vi "校准设置页.vi"() -> ()   [LabVIEW 2016]
uses:
  <vilib>/Analysis/6fits.llb/Curve Fitting Criteria.ctl
  <vilib>/Analysis/NI_AALPro.lvlib
  <vilib>/ptbypt/NI_PtbyPt.lvlib
panel:
  in  "历史数据导入":T1(radio)
  out "校准任务":bool
  in  "二次方程2":cluster{"x^2":dbl, "K":dbl, "B":dbl}
  in  "公式切换阈值滴定数(0~9999)":dbl
  out "校准状态":T2(ring)
  out "模型刷新":bool
  in  "校准按钮":T1(radio)
  in  "校准导入":bool
  in  "曲线模型":T3={"标液浓度1"=0.0, "测量吸光度1"=0.0, "样品1启用"=FALSE, "标液浓度2"=0.0, "测量吸光度2"=0.0, "样品2启用"=FALSE, "标液浓度3"=0.0, "测量吸光度3"=0.0, "样品3启用"=FALSE, "标液浓度4"=0.0, "测量吸光度4"=0.0, "样品4启用"=FALSE, "标液浓度5"=0.0, "测量吸光度5"=0.0, "样品5启用"=FALSE, "模型"=enum."线性", "精度"=4.0, "XY图"=[], "拟合公式"="", "r^2"=0.0, "标样一校准时间"=timestamp(0 s since 1904-01-01), "标样二校准时间"=timestamp(0 s since 1904-01-01), "标样三校准时间"=timestamp(0 s since 1904-01-01), "标样四校准时间"=timestamp(0 s since 1904-01-01), "标样五校准时间"=timestamp(0 s since 1904-01-01), "二次方程"={"x^2"=0.0, "K"=0.0, "B"=0.0}, "标定时间"=timestamp(0 s since 1904-01-01), "拟合公式 2"="", "r^2 2"=0.0} {"r^2 2" format="%.7f"; "标定时间" format="%<%Y/%m/%d %H:%M:%S>T"; "标样五校准时间" format="%<%Y/%m/%d %H:%M:%S>T"; "标样四校准时间" format="%<%Y/%m/%d %H:%M:%S>T"; "标样三校准时间" format="%<%Y/%m/%d %H:%M:%S>T"; "标样二校准时间" format="%<%Y/%m/%d %H:%M:%S>T"; "标样一校准时间" format="%<%Y/%m/%d %H:%M:%S>T"; "r^2" format="%.7f"; "测量吸光度5" format="%#.6f"; "测量吸光度4" format="%#.6f"; "测量吸光度3" format="%#.6f"; "测量吸光度2" format="%#.6f"; "测量吸光度1" format="%#.6f"}
  in  "测量模式":T4(ring)
  in  "参数下拉列表":u16(ring)=1 items=["挥发酚"=1]
  in  "量程下拉列表":enum16{"低量程", "高量程"}(ring)
  # "校准时间"
  # "标液浓度"
  # "滴定数"
  # "标液一"
  # "标液二"
  # "标液三"
  # "零点"
  # "跨度"
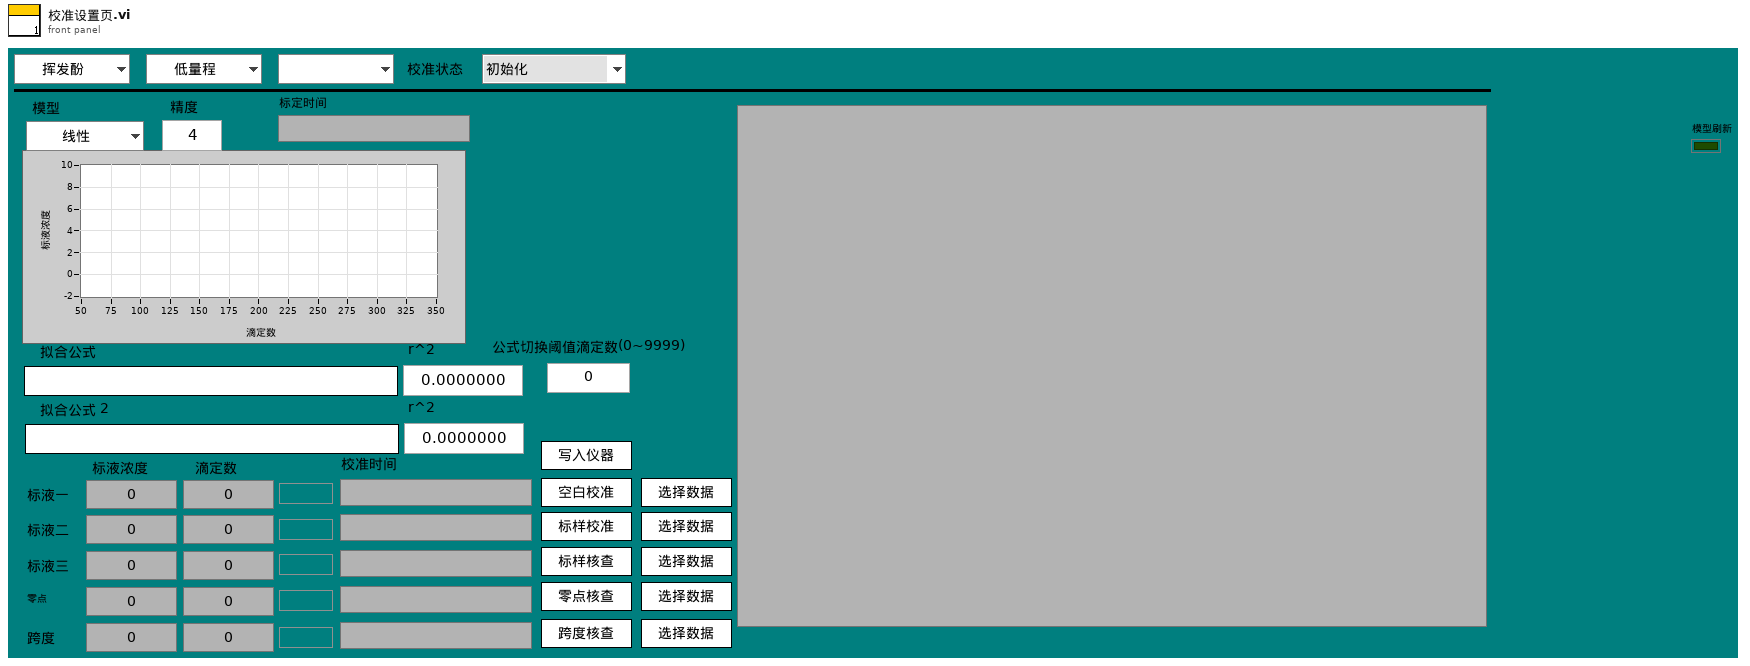
[diagram p1: front panel]
types:
  T1 = enum32{"未选择", "空白校准", "标样校准", "标样核查", "零点核查", "跨度核查"}
  T2 = enum16{"初始化", "解析数据", "判断任务类型", "执行测试任务", "等待测试任务完成", "获取测试数据", "任务结束判定", "计算公式", "结束"}
  T3 = cluster{"标液浓度1":dbl, "测量吸光度1":dbl, "样品1启用":bool, "标液浓度2":dbl, "测量吸光度2":dbl, "样品2启用":bool, "标液浓度3":dbl, "测量吸光度3":dbl, "样品3启用":bool, "标液浓度4":dbl, "测量吸光度4":dbl, "样品4启用":bool, "标液浓度5":dbl, "测量吸光度5":dbl, "样品5启用":bool, "模型":enum32{"线性", "多项式", "折线"}, "精度":dbl, "XY图":cluster{"X Values":dbl[], "Y Values":dbl[]}[], "拟合公式":string, "r^2":dbl, "标样一校准时间":timestamp, "标样二校准时间":timestamp, "标样三校准时间":timestamp, "标样四校准时间":timestamp, "标样五校准时间":timestamp, "二次方程":cluster{"x^2":dbl, "K":dbl, "B":dbl}, "标定时间":timestamp, "拟合公式 2":string, "r^2 2":dbl}
  T4 = enum16{"", "水样测量", "标样核查", "零点核查", "跨度核查", "空白测试", "平行样测试", "加标回收", "空白校准", "标样校准"}
  T5 = typedef "校准任务.ctl" = cluster{"id":u16, "任务类型":enum16{"未选择", "空白校准", "标样校准", "标样核查", "零点核查", "跨度核查"}, "量程下拉列表":enum16{"低量程", "高量程"}, "状态":enum16{"已执行", "待执行", "执行中", "停止"}, "标液浓度":dbl, "吸光值":dbl, "校准时间":timestamp, "报警状态":enum16{"正常数据", "报警数据"}}
  T6 = enum16{"", "水样测量", "标样核查", "零点核查", "跨度核查", "空白测试", "平行样测试", "加标回收"}
  T7 = cluster{"标液浓度1":dbl, "测量吸光度1":dbl, "样品1启用":bool, "标液浓度2":dbl, "测量吸光度2":dbl, "样品2启用":bool, "标液浓度3":dbl, "测量吸光度3":dbl, "样品3启用":bool, "标液浓度4":dbl, "测量吸光度4":dbl, "样品4启用":bool, "标液浓度5":dbl, "测量吸光度5":dbl, "样品5启用":bool, "模型":enum32{"线性", "多项式", "折线"}, "精度":dbl, "XY图":cluster{"X Values":dbl[], "Y Values":dbl[]}[], "拟合公式":string, "r^2":dbl, "标样一校准时间":timestamp, "标样二校准时间":timestamp, "标样三校准时间":timestamp, "标样四校准时间":timestamp, "标样五校准时间":timestamp, "二次方程":cluster{"c":dbl, "x":dbl, "x^2":dbl}, "标定时间":timestamp, "拟合公式 2":string, "r^2 2":dbl}[][]
  T8 = cluster{"标液浓度1":dbl, "测量吸光度1":dbl, "样品1启用":bool, "标液浓度2":dbl, "测量吸光度2":dbl, "样品2启用":bool, "标液浓度3":dbl, "测量吸光度3":dbl, "样品3启用":bool, "标液浓度4":dbl, "测量吸光度4":dbl, "样品4启用":bool, "标液浓度5":dbl, "测量吸光度5":dbl, "样品5启用":bool, "模型":enum32{"线性", "多项式", "折线"}, "精度":dbl, "XY图":cluster{"X Values":dbl[], "Y Values":dbl[]}[], "拟合公式":string, "r^2":dbl, "标样一校准时间":timestamp, "标样二校准时间":timestamp, "标样三校准时间":timestamp, "标样四校准时间":timestamp, "标样五校准时间":timestamp, "二次方程":cluster{"c":dbl, "x":dbl, "x^2":dbl}, "标定时间":timestamp, "拟合公式 2":string, "r^2 2":dbl}
  T9 = typedef "NI_AALPro.lvlib/Curve Fitting Criteria.ctl" = u16
  T10 = enum32{"Bad", "Idle", "Run top level", "Running"}
  T11 = cluster{"时间":timestamp, "标液值":dbl, "检测值":dbl, "吸光值":dbl}
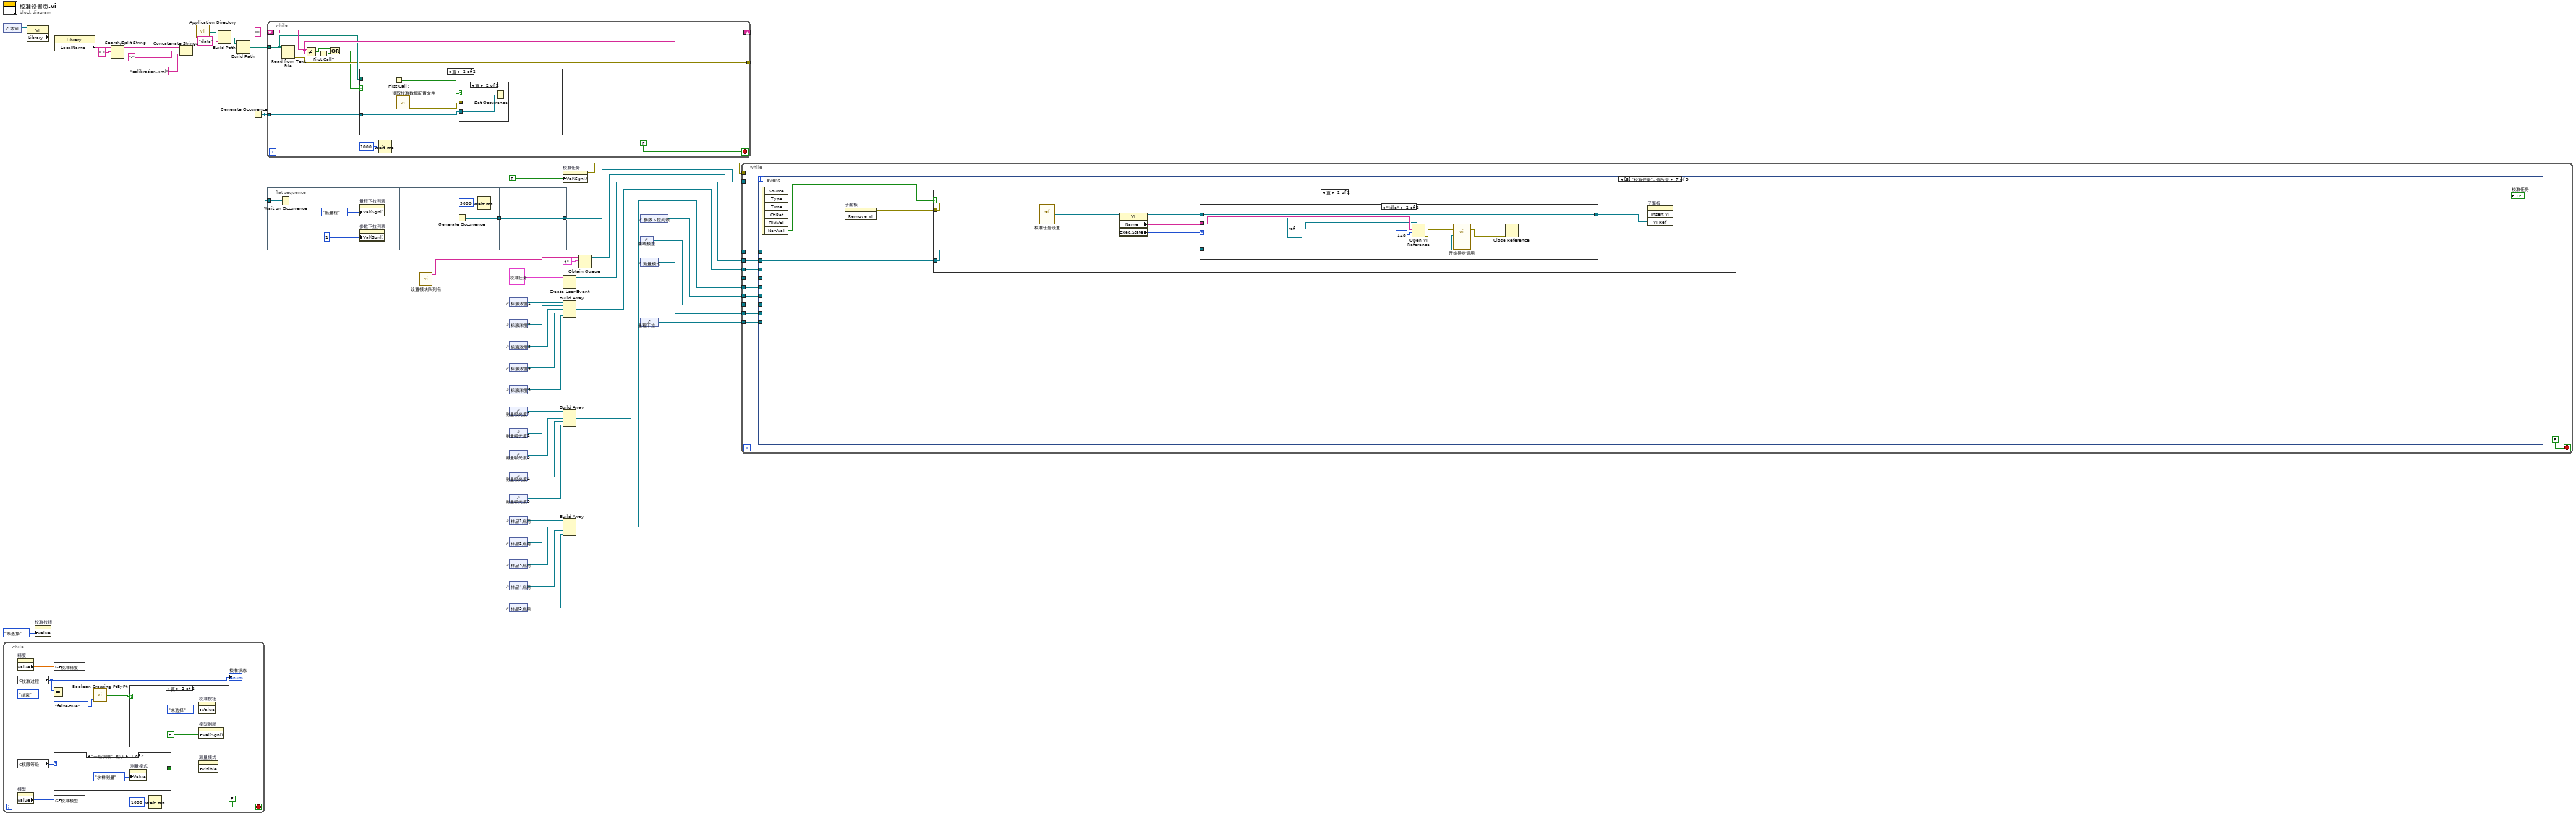
[diagram p0: block diagram]
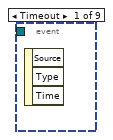
[diagram p4: hidden frame]
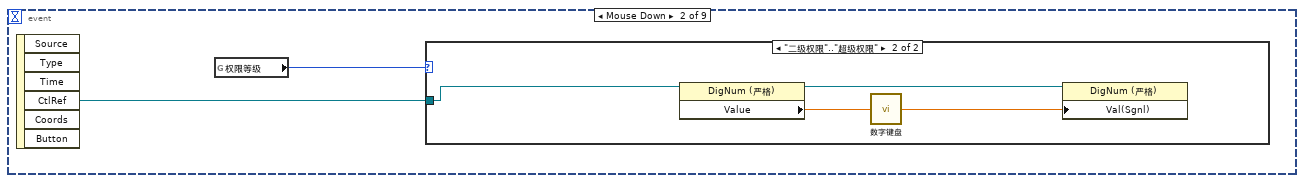
[diagram p5: hidden frame]
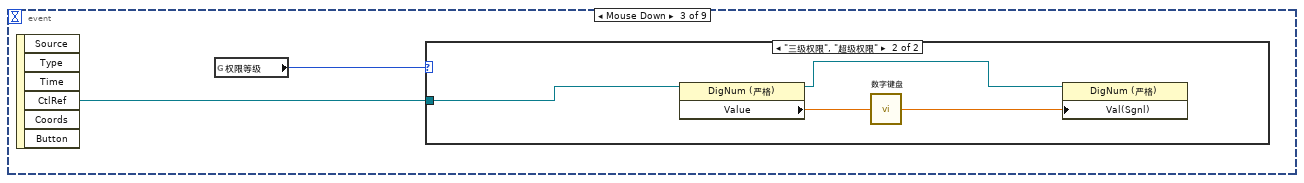
[diagram p7: hidden frame]
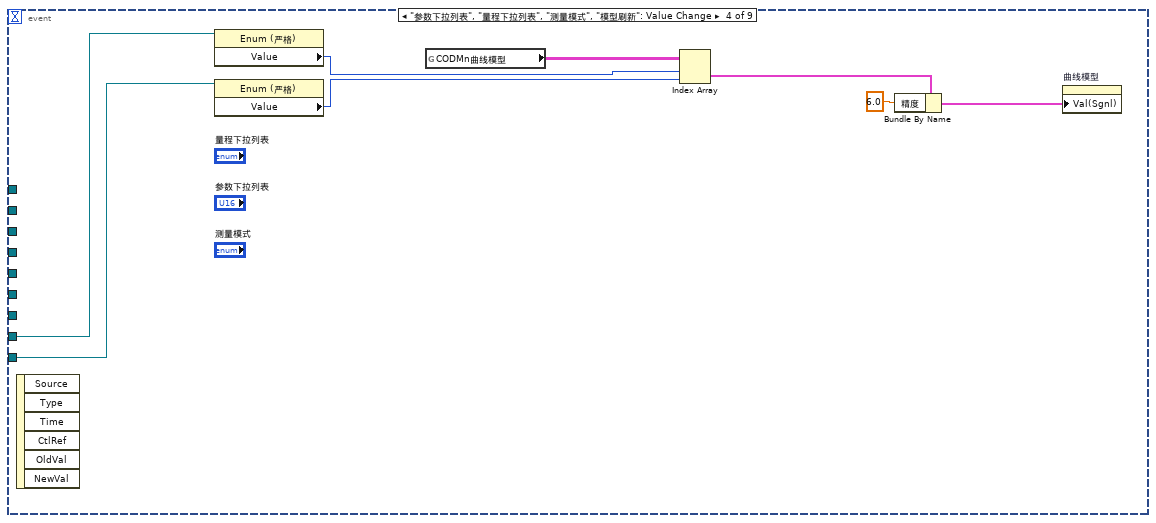
[diagram p9: hidden frame]
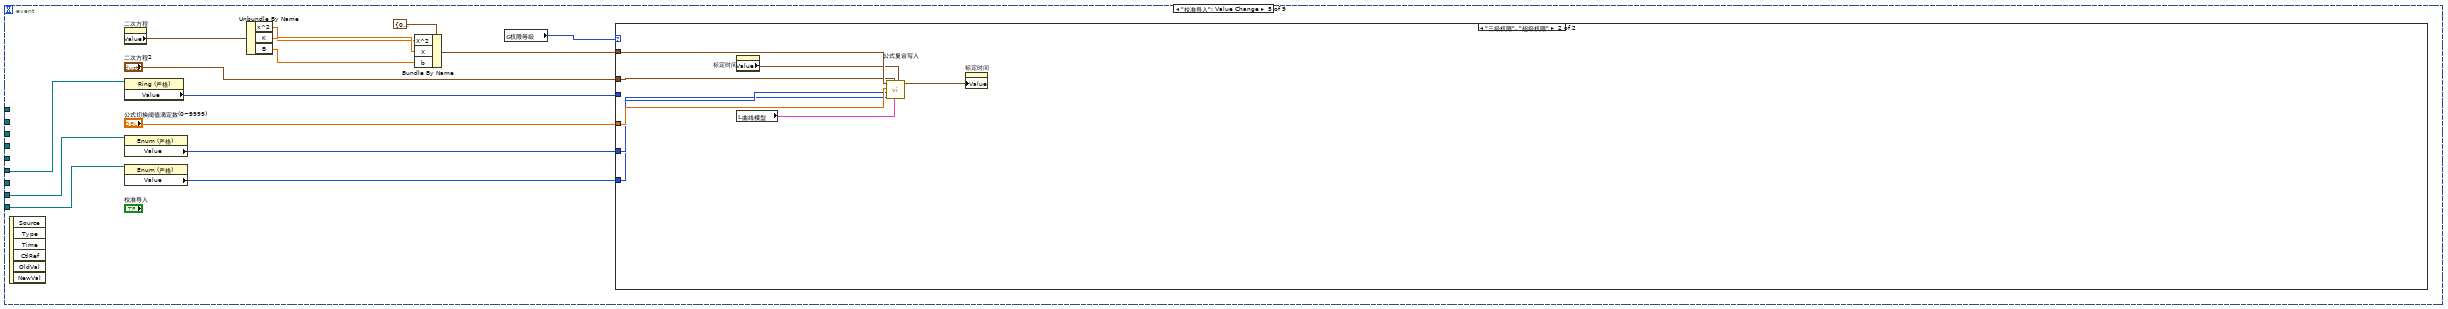
[diagram p10: hidden frame]
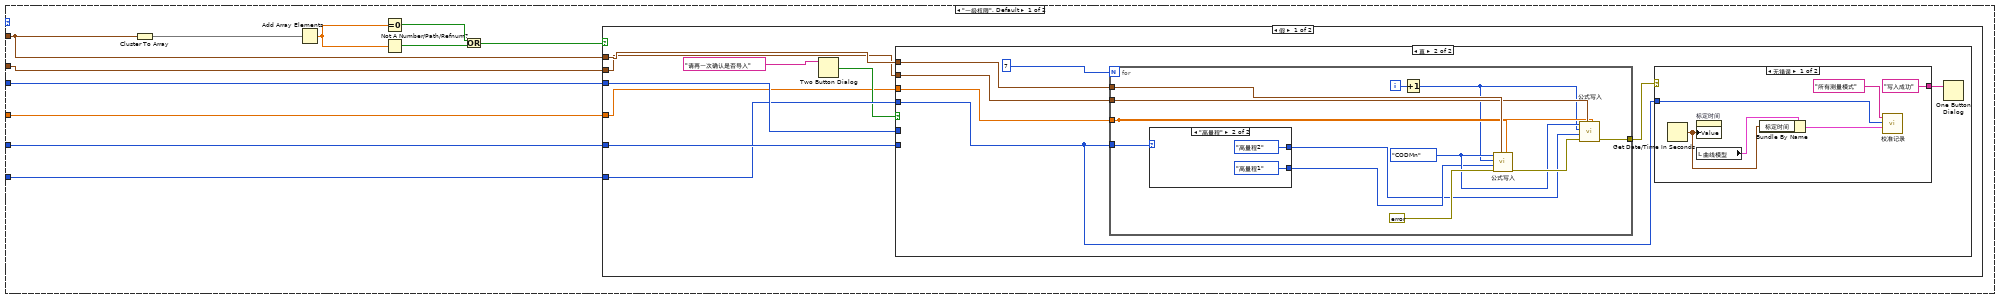
[diagram p11: hidden frame]
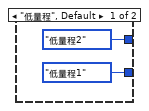
[diagram p13: hidden frame]
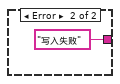
[diagram p14: hidden frame]
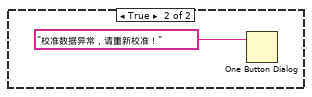
[diagram p15: hidden frame]
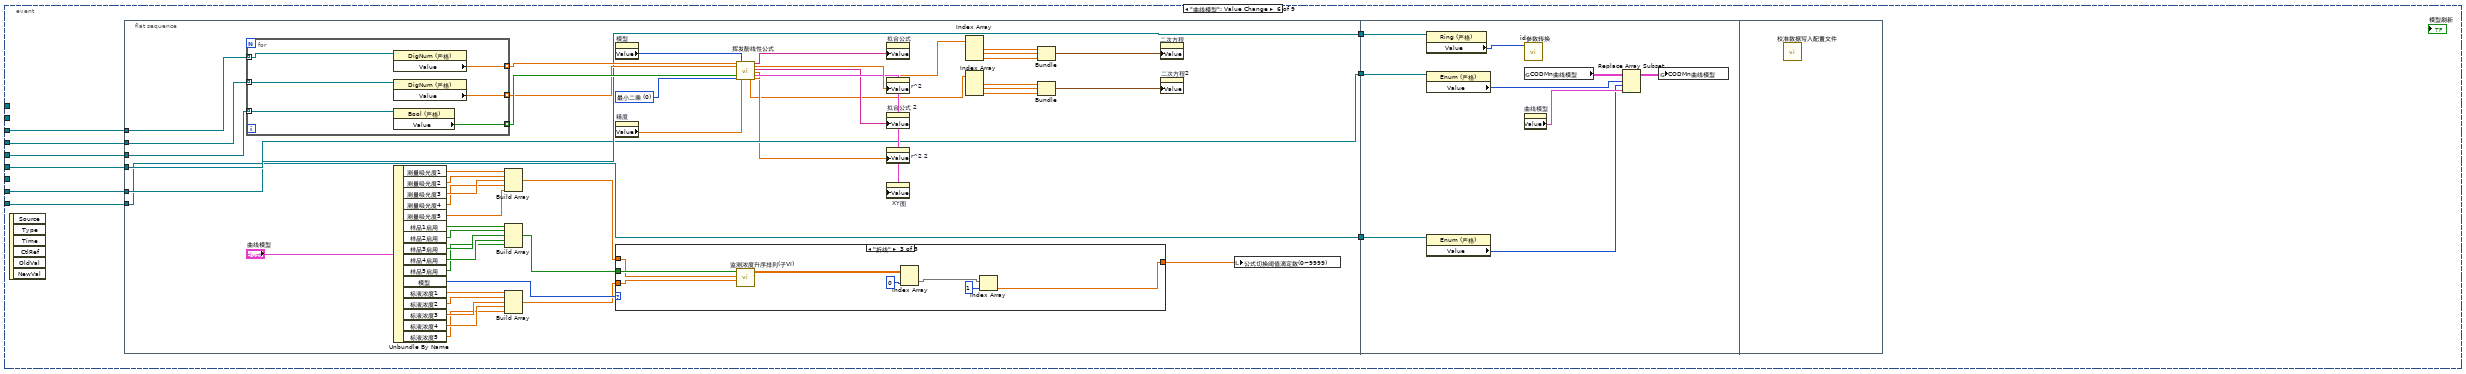
[diagram p16: hidden frame]
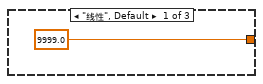
[diagram p17: hidden frame]
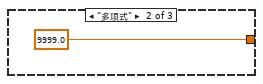
[diagram p18: hidden frame]
diagram:
  n1 = control-ref of="本VI"() -> (w8:refnum<vi>)
  n2 = while {
    stop <- FALSE stop-if-true
    n3 = property on="精度" class="DigNum (严格)"() -> ("Value"=w47:dbl)  [unwired: 2 in, 2 out]
    n4 = global read "VAR挥发酚全局变量.vi" "校准过程"() -> (w49:T2)
    "校准状态" <- w49
    n5 = global read "VAR挥发酚全局变量.vi" "权限等级"() -> (w55:enum16{"一级权限", "二级权限", "三级权限", "超级权限"})
    n6 = property on="模型" class="Enum (严格)"() -> ("Value"=w48:enum32{"线性", "多项式", "折线"})  [unwired: 2 in, 2 out]
    n7 = Equal?(x=w49, y=T2."结束" ("校准过程")) -> (x = y?=w53:bool)
    n8 = global write "VAR挥发酚全局变量.vi" "校准精度"(w47) -> ()
    n9 = case shown="\"一级权限\", 默认" w55 {
      tunnel: [_ TRUE ("可见")] -> w54
      frame "一级权限", Default {
        n10 = property on="测量模式" class="Enum (严格)"("Value"=T6."水样测量" ("测量模式")) -> ()  [unwired: 2 in, 2 out]
      }
      frame "三级权限", "超级权限" {
      }
    }
    n11 = global write "VAR挥发酚全局变量.vi" "校准模型"(w48) -> ()
    n12 = call <vilib>:"Boolean Crossing PtByPt.vi"("direction"=enum16{"either", "false-true", "true-false"}."false-true", "input"=w53) -> ("crossing"=w51:bool)  [unwired: 1 in]
    n13 = case shown="真" w51 {
      frame False {
      }
      frame True {
        n14 = property on="校准按钮" class="RadioBtnsControl (严格)"("Value"=T1."未选择" ("校准按钮")) -> ()  [unwired: 2 in, 2 out]
        n15 = property on="模型刷新" class="Bool (严格)"("Val(Sgnl)"=FALSE ("值(信号)")) -> ()  [unwired: 2 in, 2 out]
      }
    }
    n16 = Wait (ms)(milliseconds to wait=u32 1000 ("等待时间（毫秒）")) -> ()  [unwired: 1 out]
    n17 = property on="测量模式" class="Enum (严格)"("Visible"=w54) -> ()  [unwired: 2 in, 2 out]
  }
  n18 = property class="VI"(reference=w8) -> ("Library"=w17:refnum<vi>)  [unwired: 1 in, 2 out]
  n19 = property on="校准按钮" class="RadioBtnsControl (严格)"("Value"=T1."未选择" ("校准按钮")) -> ()  [unwired: 2 in, 2 out]
  n20 = property class="Library"(reference=w17) -> ("LocalName"=w15:string)  [unwired: 1 in, 2 out]
  n21 = Search/Split String(string=w15, search string/char (-)="." ("搜索字符串/字符(-)")) -> (substring before match=w13:string)  [unwired: 1 in, 2 out]
  n22 = Concatenate Strings(w13, "-" ("字符串"), "calibration.xml" ("名称或相对路径")) -> (w10:string)
  n23 = call <vilib>:"Application Directory.vi"() -> ("Application Directory"=w18:path)
  n24 = Build Path(base path=w18, name or relative path="data" ("名称或相对路径")) -> (appended path=w16:path)
  n25 = Build Path(base path=w16, name or relative path=w10) -> (appended path=w9:path)
  n26 = Generate Occurrence() -> (w6:refnum<k4>)
  n27 = while {
    shift-right: [w69] -> _
    shift-left: "" -> [w70]
    tunnel: w9 -> [w68]
    tunnel: [w66] -> _
    tunnel: w6 -> [w62]
    stop <- FALSE stop-if-true
    n28 = Read from Text File(file (use dialog)=w68) -> (text=w69:string, error out=w66:errorcluster)  [unwired: 3 in, 2 out]
    n29 = Not Equal?(x=w70, y=w69) -> (x != y?=w64:bool)
    n30 = First Call?() -> (First Call?: T/F=w65:bool)
    n31 = Or(x=w64, y=w65) -> (x .or. y?=w63:bool)
    n32 = case shown="真" w63 {
      tunnel: w68 -> [_ _]
      tunnel: w62 -> [_ w73]
      frame False {
      }
      frame True {
        n33 = First Call?() -> (First Call?: T/F=w74:bool)
        n34 = call "读取校准数据配置文件.vi"() -> ("错误输出"=w72:errorcluster)  [unwired: 11 in]
        n35 = case shown="真" w74 {
          tunnel: w73 -> [_ w75]
          tunnel: w72 -> [_ _]
          frame False {
          }
          frame True {
            n36 = Set Occurrence(w75) -> ()
          }
        }
      }
    }
    n37 = Wait (ms)(milliseconds to wait=u32 1000 ("等待时间（毫秒）")) -> ()  [unwired: 1 out]
  }
  n38 = flat-sequence {
    tunnel: w6 -> [w76]
    tunnel: [w80] -> w46
    tunnel: [w81] -> w45
    tunnel: w46 -> [w81]
    frame #0 {
      n39 = Wait on Occurrence(2:w76) -> ()  [unwired: 2 in, 1 out]
    }
    frame #1 {
      n40 = property on="量程下拉列表" class="Enum (严格)"("Val(Sgnl)"=enum16{"低量程", "高量程"}."低量程" ("值(信号)")) -> ()  [unwired: 2 in, 2 out]
      n41 = property on="参数下拉列表" class="Ring (严格)"("Val(Sgnl)"=u16 1 ("值(信号)")) -> ()  [unwired: 2 in, 2 out]
    }
    frame #2 {
      n42 = Generate Occurrence() -> (w80:refnum<k4>)
      n43 = Wait (ms)(milliseconds to wait=u32 5000 ("等待时间（毫秒）")) -> ()  [unwired: 1 out]
    }
    frame #3 {
    }
  }
  n44 = call "设置模块队列名.vi"() -> ("Msg"=w1:string)  [unwired: 11 in]
  n45 = control-ref of="标液浓度1"() -> (w31:refnum<vi>)
  n46 = control-ref of="标液浓度2"() -> (w30:refnum<vi>)
  n47 = control-ref of="标液浓度3"() -> (w29:refnum<vi>)
  n48 = control-ref of="标液浓度4"() -> (w28:refnum<vi>)
  n49 = control-ref of="标液浓度5"() -> (w27:refnum<vi>)
  n50 = control-ref of="测量吸光度1"() -> (w33:refnum<vi>)
  n51 = control-ref of="测量吸光度2"() -> (w34:refnum<vi>)
  n52 = control-ref of="测量吸光度3"() -> (w35:refnum<vi>)
  n53 = control-ref of="测量吸光度4"() -> (w36:refnum<vi>)
  n54 = control-ref of="测量吸光度5"() -> (w37:refnum<vi>)
  n55 = control-ref of="样品1启用"() -> (w43:refnum<vi>)
  n56 = control-ref of="样品2启用"() -> (w42:refnum<vi>)
  n57 = control-ref of="样品3启用"() -> (w41:refnum<vi>)
  n58 = control-ref of="样品4启用"() -> (w40:refnum<vi>)
  n59 = control-ref of="样品5启用"() -> (w39:refnum<vi>)
  n60 = property on="校准任务" class="Bool (严格)"("Val(Sgnl)"=TRUE ("值(信号)")) -> (error out=w4:errorcluster)  [unwired: 2 in, 1 out]
  n61 = Create User Event(user event datatype=T5 {"id"=0, "任务类型"=enum."未选择", "量程下拉列表"=enum."低量程", "状态"=enum."已执行", "标液浓度"=0.0, "吸光值"=0.0, "校准时间"=timestamp(0 s since 1904-01-01), "报警状态"=enum."正常数据"} ("校准任务")) -> (user event=w2:refnum<user-event>)  [unwired: 1 in, 1 out]
  n62 = Build Array(w31, w30, w29, w28, w27) -> (w26:refnum<vi>[])
  n63 = Build Array(w33, w34, w35, w36, w37) -> (w32:refnum<vi>[])
  n64 = Build Array(w43, w42, w41, w40, w39) -> (w38:refnum<vi>[])
  n65 = Obtain Queue(name (unnamed)=w1, element data type=cluster{"命令":string, "data":variant} {"命令"="", "data"=variant}) -> (queue out=w22:refnum<queue>)  [unwired: 3 in, 2 out]
  n66 = control-ref of="参数下拉列表"() -> (w44:refnum<vi>)
  n67 = control-ref of="曲线模型"() -> (w20:refnum<vi>)
  n68 = control-ref of="测量模式"() -> (w25:refnum<vi>)
  n69 = control-ref of="量程下拉列表"() -> (w24:refnum<vi>)
  n70 = while {
    tunnel: w45 -> [_]
    tunnel: w44 -> [w90]
    tunnel: w38 -> [w89]
    tunnel: w32 -> [w88]
    tunnel: w26 -> [w87]
    tunnel: w25 -> [w86]
    tunnel: w24 -> [w85]
    tunnel: w22 -> [w84]
    tunnel: w20 -> [w83]
    tunnel: w4 -> [_]
    tunnel: w2 -> [w82]
    stop <- FALSE stop-if-true
    n71 = event shown="[6] \"校准任务\": 值改变" {
      selector: _ -> [_ _ _ _ _ _ _ _ _]
      dyn-events: _ -> [_ _ _ _ _ _ _ _ _]
      timeout: _ -> [_ _ _ _ _ _ _ _ _]
      tunnel: w90 -> [_ _ _ _ w126 w189 _ w295 w323]
      tunnel: w89 -> [_ _ _ _ _ w193 _ _ _]
      tunnel: w88 -> [_ _ _ _ _ w192 _ _ _]
      tunnel: w87 -> [_ _ _ _ _ w191 _ _ _]
      tunnel: w86 -> [_ _ _ w111 w124 w187 _ w290 w318]
      tunnel: w85 -> [_ _ _ w110 w122 w185 _ w294 w322]
      tunnel: w84 -> [_ _ _ _ _ _ _ w296 w324]
      tunnel: w83 -> [_ _ _ _ _ _ _ w288 _]
      tunnel: w82 -> [_ _ _ _ _ _ w268 w287 w317]
      event Timeout {
        n72 = event-data() -> ()  [unwired: 1 in, 3 out]
      }
      event "曲线模型.标液浓度1", "曲线模型.标液浓度2", "曲线模型.标液浓度3", "曲线模型.标液浓度4", "曲线模型.标液浓度5", "曲线模型.精度": Mouse Down {
        n73 = event-data() -> ("CtlRef"=w93:refnum<vi>)  [unwired: 1 in, 5 out]
        n74 = global read "VAR挥发酚全局变量.vi" "权限等级"() -> (w92:enum16{"一级权限", "二级权限", "三级权限", "超级权限"})
        n75 = case shown="\"二级权限\"..\"超级权限\"" w92 {
          tunnel: w93 -> [_ w97]
          frame "一级权限", Default {
          }
          frame "二级权限".."超级权限" {
            n76 = property class="DigNum (严格)"(reference=w97) -> (reference out=w95:refnum<vi>, "Value"=w96:dbl)  [unwired: 1 in, 1 out]
            n77 = call "数字键盘.vi"("OldNumber"=w96) -> ("NewNumber"=w94:dbl)
            n78 = property class="DigNum (严格)"(reference=w95, "Val(Sgnl)"=w94) -> ()  [unwired: 1 in, 2 out]
          }
        }
      }
      event "曲线模型.测量吸光度1", "曲线模型.测量吸光度2", "曲线模型.测量吸光度3", "曲线模型.测量吸光度4", "曲线模型.测量吸光度5": Mouse Down {
        n79 = event-data() -> ("CtlRef"=w99:refnum<vi>)  [unwired: 1 in, 5 out]
        n80 = global read "VAR挥发酚全局变量.vi" "权限等级"() -> (w98:enum16{"一级权限", "二级权限", "三级权限", "超级权限"})
        n81 = case shown="\"三级权限\", \"超级权限\"" w98 {
          tunnel: w99 -> [_ w103]
          frame "一级权限", Default {
          }
          frame "三级权限", "超级权限" {
            n82 = property class="DigNum (严格)"(reference=w103) -> (reference out=w101:refnum<vi>, "Value"=w102:dbl)  [unwired: 1 in, 1 out]
            n83 = call "数字键盘.vi"("OldNumber"=w102) -> ("NewNumber"=w100:dbl)
            n84 = property class="DigNum (严格)"(reference=w101, "Val(Sgnl)"=w100) -> ()  [unwired: 1 in, 2 out]
          }
        }
      }
      event "参数下拉列表", "量程下拉列表", "测量模式", "模型刷新": Value Change {
        n85 = event-data() -> ()  [unwired: 1 in, 6 out]
        n86 = property class="Enum (严格)"(reference=w111) -> ("Value"=w108:T4)  [unwired: 1 in, 2 out]
        n87 = property class="Enum (严格)"(reference=w110) -> ("Value"=w107:enum16{"低量程", "高量程"})  [unwired: 1 in, 2 out]
        n88 = global read "校准数据全局变量.vi" "CODMn曲线模型"() -> (w109:T7)
        n89 = Index Array(array=w109, index (row)=w108, index (col)=w107) -> (element=w106:T8)
        n90 = Bundle By Name(cluster=w106, "精度"=6.0 ("值")) -> (w105:T8)
        n91 = property on="曲线模型" class="Clust (严格)"("Val(Sgnl)"=w105) -> ()  [unwired: 2 in, 2 out]
      }
      event "校准导入": Value Change {
        n92 = event-data() -> ()  [unwired: 1 in, 6 out]
        n93 = property on="二次方程" class="Clust (严格)"() -> ("Value"=w116:cluster{"x^2":dbl, "K":dbl, "B":dbl})  [unwired: 2 in, 2 out]
        n94 = property class="Ring (严格)"(reference=w126) -> ("Value"=w125:u16)  [unwired: 1 in, 2 out]
        n95 = property class="Enum (严格)"(reference=w124) -> ("Value"=w123:T4)  [unwired: 1 in, 2 out]
        n96 = property class="Enum (严格)"(reference=w122) -> ("Value"=w121:enum16{"低量程", "高量程"})  [unwired: 1 in, 2 out]
        n97 = Unbundle By Name(w116) -> ("x^2"=w117:dbl, "K"=w118:dbl, "B"=w119:dbl)
        n98 = Bundle By Name(cluster=cluster{"X^2":dbl, "X":dbl, "b":dbl} {"X^2"=0.0, "X"=0.0, "b"=0.0} ("公式"), "X^2"=w117, "X"=w118, "b"=w119) -> (w115:cluster{"X^2":dbl, "X":dbl, "b":dbl})
        n99 = global read "VAR挥发酚全局变量.vi" "权限等级"() -> (w120:enum16{"一级权限", "二级权限", "三级权限", "超级权限"})
        n100 = case shown="\"三级权限\", \"超级权限\"" w120 {
          tunnel: w125 -> [w137 _]
          tunnel: w123 -> [w136 w182]
          tunnel: w121 -> [w135 w181]
          tunnel: w115 -> [w129 w184]
          tunnel: "公式切换阈值滴定数(0~9999)" -> [w128 w183]
          tunnel: "二次方程2" -> [w127 w180]
          frame "一级权限", Default {
            n101 = Cluster To Array(cluster=w129) -> (array=w134:dbl[])
            n102 = Add Array Elements(numeric array=w134) -> (sum=w133:dbl)
            n103 = Equal To 0?(x=w133) -> (x = 0?=w131:bool)
            n104 = Not A Number/Path/Refnum?(number/path/refnum=w133) -> (NaN/Path/Refnum?=w132:bool)
            n105 = Or(x=w131, y=w132) -> (x .or. y?=w130:bool)
            n106 = case shown="假" w130 {
              tunnel: w137 -> [w145 _]
              tunnel: w136 -> [w144 _]
              tunnel: w135 -> [w143 _]
              tunnel: w129 -> [w140 _]
              tunnel: w128 -> [w139 _]
              tunnel: w127 -> [w138 _]
              frame False {
                n107 = Two Button Dialog(message="请再一次确认是否导入" ("消息")) -> (T button?=w141:bool)  [unwired: 2 in]
                n108 = case shown="真" w141 {
                  tunnel: w145 -> [_ _]
                  tunnel: w144 -> [_ _]
                  tunnel: w143 -> [_ w146]
                  tunnel: w140 -> [_ w151]
                  tunnel: w139 -> [_ w148]
                  tunnel: w138 -> [_ w149]
                  frame False {
                  }
                  frame True {
                    n109 = for {
                      N: 7 -> [_]
                      tunnel: w151 -> [w163]
                      tunnel: [w161] -> w150
                      tunnel: w149 -> [w160]
                      tunnel: w148 -> [w159]
                      tunnel: w146 -> [w157]
                      i -> [w154]
                      w158 = enum16{"CODMn"}."CODMn" ("测量参数")
                      n110 = case shown="\"高量程\"" w157 {
                        tunnel: [enum16{"低量程1", "低量程2", "高量程1", "高量程2"}."低量程1" ("量程") enum16{"低量程1", "低量程2", "高量程1", "高量程2"}."高量程1" ("量程")] -> w156
                        tunnel: [enum16{"低量程1", "低量程2", "高量程1", "高量程2"}."低量程2" ("量程") enum16{"低量程1", "低量程2", "高量程1", "高量程2"}."高量程2" ("量程")] -> w155
                        frame "低量程", Default {
                        }
                        frame "高量程" {
                        }
                      }
                      n111 = Increment(x=w154) -> (x+1=w153:i32)
                      n112 = call "公式写入.vi"("临界滴定数"=w159, "公式"=w163, "error in (no error)"=errorcluster {"status"=FALSE, "code"=0, "source"=""} ("error out"), "量程"=w156, "测量模式"=w153, "测量参数"=w158) -> ("error out"=w162:errorcluster)  [unwired: 5 in]
                      n113 = call "公式写入.vi"("临界滴定数"=w159, "公式"=w160, "error in (no error)"=w162, "量程"=w155, "测量模式"=w153, "测量参数"=w158) -> ("error out"=w161:errorcluster)  [unwired: 5 in]
                    }
                    n114 = case shown="无错误" w150 {
                      tunnel: ["写入成功" "写入失败"] -> w152
                      tunnel: w146 -> [w173 _]
                      frame No Error {
                        n115 = Get Date/Time In Seconds() -> (seconds since 1Jan1904=w170:timestamp)
                        n116 = property on="标定时间" class="AbsTime (严格)"("Value"=w170) -> ()  [unwired: 2 in, 2 out]
                        n117 = local read "曲线模型"() -> (w171:T3)
                        n118 = Bundle By Name(cluster=w171, "标定时间"=w170) -> (w169:T3)
                        n119 = call "校准记录.vi"("曲线模型"=w169, "量程"=w173, "测量模式"="所有测量模式") -> ()  [unwired: 8 in, 1 out]
                      }
                      frame Error {
                      }
                    }
                    n120 = One Button Dialog(message=w152) -> ()  [unwired: 1 in, 1 out]
                  }
                }
              }
              frame True {
                n121 = One Button Dialog(message="校准数据异常，请重新校准！" ("消息")) -> ()  [unwired: 1 in, 1 out]
              }
            }
          }
          frame "三级权限", "超级权限" {
            n122 = property on="标定时间" class="AbsTime (严格)"() -> ("Value"=w177:timestamp)  [unwired: 2 in, 2 out]
            n123 = local read "曲线模型"() -> (w178:T3)
            n124 = call "公式复合写入.vi"("标定时间输入"=w177, "曲线模型"=w178, "公式 2"=w180, "量程下拉列表"=w181, "测量模式"=w182, "临界滴定数"=w183, "公式"=w184) -> ("标定时间输出"=w179:timestamp)  [unwired: 4 in]
            n125 = property on="标定时间" class="AbsTime (严格)"("Value"=w179) -> ()  [unwired: 2 in, 2 out]
          }
        }
      }
      event "曲线模型": Value Change {
        n126 = event-data() -> ()  [unwired: 1 in, 6 out]
        n127 = flat-sequence {
          tunnel: w193 -> [w241]
          tunnel: w192 -> [w239]
          tunnel: w191 -> [w237]
          tunnel: [w224] -> w190
          tunnel: w189 -> [w224]
          tunnel: [w223] -> w188
          tunnel: w187 -> [w223]
          tunnel: [w222] -> w186
          tunnel: w185 -> [w222]
          tunnel: w190 -> [w266]
          tunnel: w188 -> [w263]
          tunnel: w186 -> [w262]
          frame #0 {
            w233 = T9 0 items=["最小二乘", "最小绝对残差", "Bisquare"] ("method")
            n128 = for {
              tunnel: w241 -> [w257] mode=indexing
              tunnel: [w256] -> w240 mode=indexing
              tunnel: w239 -> [w255] mode=indexing
              tunnel: [w254] -> w238 mode=indexing
              tunnel: w237 -> [w253] mode=indexing
              tunnel: [w252] -> w236 mode=indexing
              n129 = property class="DigNum (严格)"(reference=w253) -> ("Value"=w252:dbl)  [unwired: 1 in, 2 out]
              n130 = property class="DigNum (严格)"(reference=w255) -> ("Value"=w254:dbl)  [unwired: 1 in, 2 out]
              n131 = property class="Bool (严格)"(reference=w257) -> ("Value"=w256:bool)  [unwired: 1 in, 2 out]
            }
            n132 = Unbundle By Name("曲线模型") -> ("测量吸光度1"=w220:dbl, "测量吸光度2"=w219:dbl, "测量吸光度3"=w218:dbl, "测量吸光度4"=w216:dbl, "测量吸光度5"=w217:dbl, "样品1启用"=w215:bool, "样品2启用"=w214:bool, "样品3启用"=w213:bool, "样品4启用"=w212:bool, "样品5启用"=w211:bool, "模型"=w200:enum32{"线性", "多项式", "折线"}, "标液浓度1"=w199:dbl, "标液浓度2"=w198:dbl, "标液浓度3"=w197:dbl, "标液浓度4"=w196:dbl, "标液浓度5"=w195:dbl)
            n133 = Build Array(w220, w219, w218, w216, w217) -> (w209:dbl[])
            n134 = Build Array(w215, w214, w213, w212, w211) -> (w210:bool[])
            n135 = Build Array(w199, w198, w197, w196, w195) -> (w194:dbl[])
            n136 = property on="模型" class="Enum (严格)"() -> ("Value"=w235:enum32{"线性", "多项式", "折线"})  [unwired: 2 in, 2 out]
            n137 = property on="精度" class="DigNum (严格)"() -> ("Value"=w234:dbl)  [unwired: 2 in, 2 out]
            n138 = case shown="\"折线\"" w200 {
              tunnel: w210 -> [_ _ w249]
              tunnel: w209 -> [_ _ w248]
              tunnel: [9999.0 ("数值") 9999.0 ("数值") w250] -> w201
              tunnel: w194 -> [_ _ w247]
              frame "线性", Default {
              }
              frame "多项式" {
              }
              frame "折线" {
                n139 = call "监测浓度升序排列(子VI).vi"("标液浓度"=w247, "信号值"=w248, "启用"=w249) -> ("输出数组"=w246:dbl[][])  [unwired: 8 in]
                n140 = Index Array(array=w246, index (col)=0 ("禁用的索引 (列)")) -> (element=w244:dbl[])  [unwired: 1 in]
                n141 = Index Array(array=w244, index=1 ("索引")) -> (element=w250:dbl)
              }
            }
            n142 = call "挥发酚线性公式.vi"("标液浓度"=w236, "信号值"=w238, "启用"=w240, "method"=w233, "模型"=w235, "精度"=w234) -> ("Polynomial Coefficients 2"=w203:dbl[], "拟合方程"=w232:string, "r^2"=w231:dbl, "拟合方程 2"=w208:string, "r^2 2"=w207:dbl, "XY图"=w230:cluster{"X Values":dbl[], "Y Values":dbl[]}[], "Polynomial Coefficients"=w229:dbl[])  [unwired: 7 in]
            n143 = property on="拟合公式" class="Str"("Value"=w232) -> ()  [unwired: 2 in, 2 out]
            n144 = property on="r^2" class="DigNum (严格)"("Value"=w231) -> ()  [unwired: 2 in, 2 out]
            n145 = property on="拟合公式 2" class="Str"("Value"=w208) -> ()  [unwired: 2 in, 2 out]
            n146 = property on="r^2 2" class="DigNum (严格)"("Value"=w207) -> ()  [unwired: 2 in, 2 out]
            n147 = property on="XY图" class="XYGraph (严格)"("Value"=w230) -> ()  [unwired: 2 in, 2 out]
            n148 = Index Array(array=w229) -> (element #1=w228:dbl, element #2=w227:dbl, element #3=w226:dbl)  [unwired: 3 in]
            n149 = Index Array(array=w203) -> (element #1=w204:dbl, element #2=w205:dbl, element #3=w206:dbl)  [unwired: 3 in]
            n150 = Bundle("数值"=w228, "数值"=w227, "数值"=w226) -> (w225:cluster{"数值":dbl, "数值":dbl, "数值":dbl})  [unwired: 1 in]
            n151 = Bundle("数值"=w204, "数值"=w205, "数值"=w206) -> (w202:cluster{"数值":dbl, "数值":dbl, "数值":dbl})  [unwired: 1 in]
            n152 = property on="二次方程" class="Clust (严格)"("Value"=w225) -> ()  [unwired: 2 in, 2 out]
            n153 = property on="二次方程2" class="Clust (严格)"("Value"=w202) -> ()  [unwired: 2 in, 2 out]
            n154 = local write "公式切换阈值滴定数(0~9999)"(w201) -> ()
          }
          frame #1 {
            n155 = property class="Ring (严格)"(reference=w266) -> ("Value"=w265:u16)  [unwired: 1 in, 2 out]
            n156 = property class="Enum (严格)"(reference=w263) -> ("Value"=w260:T4)  [unwired: 1 in, 2 out]
            n157 = property class="Enum (严格)"(reference=w262) -> ("Value"=w261:enum16{"低量程", "高量程"})  [unwired: 1 in, 2 out]
            n158 = call "id参数转换.vi"("id"=w265) -> ()  [unwired: 10 in, 1 out]
            n159 = global read "校准数据全局变量.vi" "CODMn曲线模型"() -> (w259:T7)
            n160 = property on="曲线模型" class="Clust (严格)"() -> ("Value"=w264:T3)  [unwired: 2 in, 2 out]
            n161 = Replace Array Subset(array=w259, new element=w264, index (row)=w260, index (col)=w261) -> (w258:T7)
            n162 = global write "校准数据全局变量.vi" "CODMn曲线模型"(w258) -> ()
          }
          frame #2 {
            n163 = call "校准数据写入配置文件.vi"() -> ()  [unwired: 11 in, 1 out]
          }
        }
      }
      event "校准任务": Value Change {
        n164 = event-data() -> ("NewVal"=w269:bool)  [unwired: 1 in, 5 out]
        n165 = invoke on="子面板" class="SubPnl" method="Remove VI"() -> (error out=w267:errorcluster)  [unwired: 3 in, 2 out]
        n166 = case shown="真" w269 {
          tunnel: w268 -> [_ w273]
          tunnel: w267 -> [_ w270]
          frame False {
          }
          frame True {
            n167 = vi-ref "校准任务设置.vi"() -> (w276:refnum<vi>)
            n168 = property class="VI"(reference=w276) -> (reference out=w272:refnum<vi>, "Name"=w274:string, "Exec.State"=w275:T10)  [unwired: 1 in, 1 out]
            n169 = case shown="\"Idle\"" w275 {
              tunnel: w274 -> [_ w286]
              tunnel: w273 -> [_ w281]
              tunnel: w272 -> [w277 w278]
              tunnel: [w277 w278] -> w271
              frame "Bad", Default {
              }
              frame "Idle" {
                n170 = Open VI Reference(type specifier VI Refnum (for type only)=refnum<vi> refnum ("类型说明符VI引用句柄（仅用于类型）"), vi path=w286, options=128 ("选项")) -> (vi reference=w283:refnum<vi>, error out=w282:errorcluster)  [unwired: 3 in]
                n171 = call-by-ref "开始异步调用"(reference=w283, error in=w282, "用户事件"=w281) -> (reference out=w280:refnum<vi>, error out=w279:errorcluster)  [unwired: 11 in]
                n172 = Close Reference(reference=w280, error in (no error)=w279) -> ()  [unwired: 1 out]
              }
            }
            n173 = invoke on="子面板" class="SubPnl" method="Insert VI"(error in=w270, "VI Ref"=w271) -> ()  [unwired: 2 in, 4 out]
          }
        }
      }
      event "校准按钮": Value Change {
        n174 = event-data() -> ("CtlRef"=w289:refnum<vi>, "NewVal"=w291:T1)  [unwired: 1 in, 4 out]
        n175 = Not Equal?(x=w291, y=T1."未选择") -> (x != y?=w292:bool)
        n176 = case shown="真" w292 {
          tunnel: w296 -> [_ _]
          tunnel: w295 -> [_ w304]
          tunnel: w294 -> [_ w302]
          tunnel: w291 -> [_ w306]
          tunnel: w290 -> [_ _]
          tunnel: w289 -> [_ _]
          tunnel: w288 -> [_ _]
          tunnel: w287 -> [_ w305]
          frame False {
          }
          frame True {
            (unwired) u16 21 items=["CODMn"=21] ("参数下拉列表")
            n177 = property class="Ring (严格)"(reference=w304) -> ("Value"=w303:u16)  [unwired: 1 in, 2 out]
            n178 = property class="Enum (严格)"(reference=w302) -> ("Value"=w301:enum16{"低量程", "高量程"})  [unwired: 1 in, 2 out]
            n179 = local read "曲线模型"() -> (w299:T3)
            n180 = case shown="\"空白校准\"" w306 {
              tunnel: w299 -> [_ w308 w310 w311 w313 w315]
              tunnel: [_ w307 w309 w312 w314 w316] -> w298
              frame "未选择", Default {
              }
              frame "空白校准" {
                n181 = Unbundle By Name(w308) -> ("标液浓度1"=w307:dbl)
              }
              frame "标样校准" {
                n182 = Unbundle By Name(w310) -> ("标液浓度2"=w309:dbl)
              }
              frame "标样核查" {
                n183 = Unbundle By Name(w311) -> ("标液浓度3"=w312:dbl)
              }
              frame "零点核查" {
                n184 = Unbundle By Name(w313) -> ("标液浓度4"=w314:dbl)
              }
              frame "跨度核查" {
                n185 = Unbundle By Name(w315) -> ("标液浓度5"=w316:dbl)
              }
            }
            n186 = Bundle By Name(cluster=T5 {"id"=0, "任务类型"=enum."未选择", "量程下拉列表"=enum."低量程", "状态"=enum."待执行", "标液浓度"=0.0, "吸光值"=0.0, "校准时间"=timestamp(0 s since 1904-01-01), "报警状态"=enum."正常数据"} ("校准任务"), "id"=w303, "任务类型"=w306, "量程下拉列表"=w301, "标液浓度"=w298) -> (w300:T5)
            n187 = Generate User Event(user event=w305, event data cluster=w300) -> ()  [unwired: 2 in, 2 out]
          }
        }
      }
      event "历史数据导入": Value Change {
        n188 = event-data() -> ("NewVal"=w319:T1)  [unwired: 1 in, 5 out]
        n189 = Not Equal?(x=w319, y=T1."未选择") -> (x != y?=w320:bool)
        n190 = case shown="真" w320 {
          tunnel: w324 -> [_ _]
          tunnel: w323 -> [_ w334]
          tunnel: w322 -> [_ w333]
          tunnel: w319 -> [_ w325]
          tunnel: w318 -> [_ _]
          tunnel: w317 -> [_ w329]
          frame False {
          }
          frame True {
            n191 = property class="Ring (严格)"(reference=w334) -> ("Value"=w328:u16)  [unwired: 1 in, 2 out]
            n192 = property class="Enum (严格)"(reference=w333) -> ("Value"=w327:enum16{"低量程", "高量程"})  [unwired: 1 in, 2 out]
            n193 = property on="历史数据导入" class="RadioBtnsControl (严格)"("Value"=T1."未选择" ("历史数据导入")) -> ()  [unwired: 2 in, 2 out]
            n194 = call "id参数转换.vi"("id"=w328) -> ("table输出"=w332:string)  [unwired: 10 in]
            n195 = call "校准数据选择表.vi"("历史数据导入"=w325, "量程下拉列表"=w327, "table"=w332) -> ("布尔"=w331:bool, "输出"=w330:T11)  [unwired: 7 in]
            n196 = case shown="真" w331 {
              tunnel: w330 -> [_ w340]
              tunnel: w329 -> [_ w344]
              tunnel: w328 -> [_ w341]
              tunnel: w327 -> [_ w339]
              tunnel: w325 -> [_ w338]
              frame False {
              }
              frame True {
                n197 = Unbundle By Name(w340) -> ("标液值"=w337:dbl, "吸光值"=w336:dbl, "时间"=w335:timestamp)
                n198 = Bundle By Name(cluster=T5 {"id"=0, "任务类型"=enum."未选择", "量程下拉列表"=enum."低量程", "状态"=enum."已执行", "标液浓度"=0.0, "吸光值"=0.0, "校准时间"=timestamp(0 s since 1904-01-01), "报警状态"=enum."正常数据"} ("事件数据"), "id"=w341, "任务类型"=w338, "量程下拉列表"=w339, "标液浓度"=w337, "吸光值"=w336, "校准时间"=w335) -> (w342:T5)
                n199 = Generate User Event(user event=w344, event data cluster=w342) -> ()  [unwired: 2 in, 2 out]
              }
            }
          }
        }
      }
    }
  }
